vi "GEOM_CorrectAmplifiers.vi"(7 "BinCorrectionType":T1(ring), 8 "error in (no error)":errorcluster, 9 "modifiers":T6={"Binning"={"x"=1, "y"=1}, "sections"=[]} {"Binning"."y" min=1; "Binning"."x" min=1}, 10 "Amplifiers":T2[](array[typedef]) {"fliped" items=["none", "horizontal", "vertical"]; "type" items=["LL", "LR", "UL", "UR"]}) -> (0 "error out":errorcluster, 1 "NonBinnedAmplifiers":T2[](array[typedef]) {"fliped" items=["none", "horizontal", "vertical"]; "type" items=["LL", "LR", "UL", "UR"]}, 2 "BinnedAmplifiers":T2[](array[typedef]) {"fliped" items=["none", "horizontal", "vertical"]; "type" items=["LL", "LR", "UL", "UR"]})   [LabVIEW 2016]
uses:
  GEOM_AmpModifiers.ctl
  GEOM_Binning.ctl
  GEOM_Moifier.ctl
  GEOM_Amplifier.ctl
  GEOM_AmpType.ctl
  GEOM_ROI.ctl
  GEOM_Coords.ctl
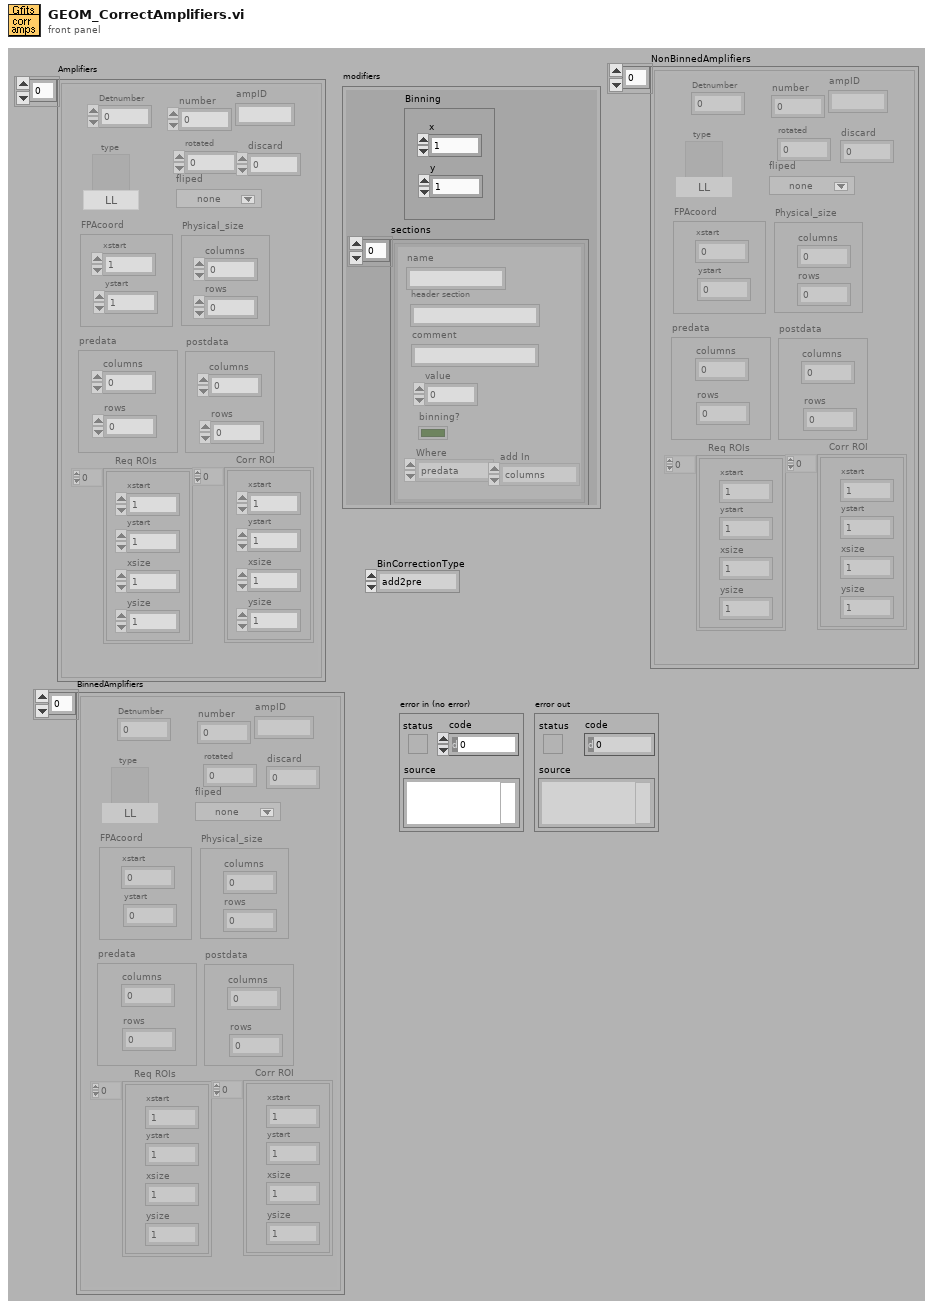
[diagram p1: front panel]
types:
  T1 = enum16{"add2pre", "add2post", "add2data", "none"}
  T2 = typedef "GEOM_Amplifier.ctl" = cluster{"number":i32, "type":T3, "rotated":i16, "fliped":u16, "FPAcoord":cluster{"xstart":i32, "ystart":i32}, "Physical_size":cluster{"columns":i32, "rows":i32}, "predata":cluster{"columns":i32, "rows":i32}, "postdata":cluster{"columns":i32, "rows":i32}, "Req ROIs":T4, "Corr ROI":T4, "Detnumber":i32, "ampID":string, "discard":i32}
  T3 = typedef "GEOM_AmpType.ctl" = u16
  T4 = typedef "GEOM_ROI.ctl" = T5[]
  T5 = typedef "GEOM_Coords.ctl" = cluster{"xstart":u32, "ystart":u32, "xsize":u32, "ysize":u32}
  T6 = typedef "GEOM_AmpModifiers.ctl" = cluster{"Binning":T7, "sections":T8[]}
  T7 = typedef "GEOM_Binning.ctl" = cluster{"x":u32, "y":u32}
  T8 = typedef "GEOM_Moifier.ctl" = cluster{"name":string, "header section":string, "comment":string, "value":i32, "binning?":bool, "Where":enum16{"predata", "postdata"}, "add In":enum16{"columns", "rows", "none"}}
  T9 = cluster{"xstart":i32, "ystart":i32, "columns":i32, "rows":i32}
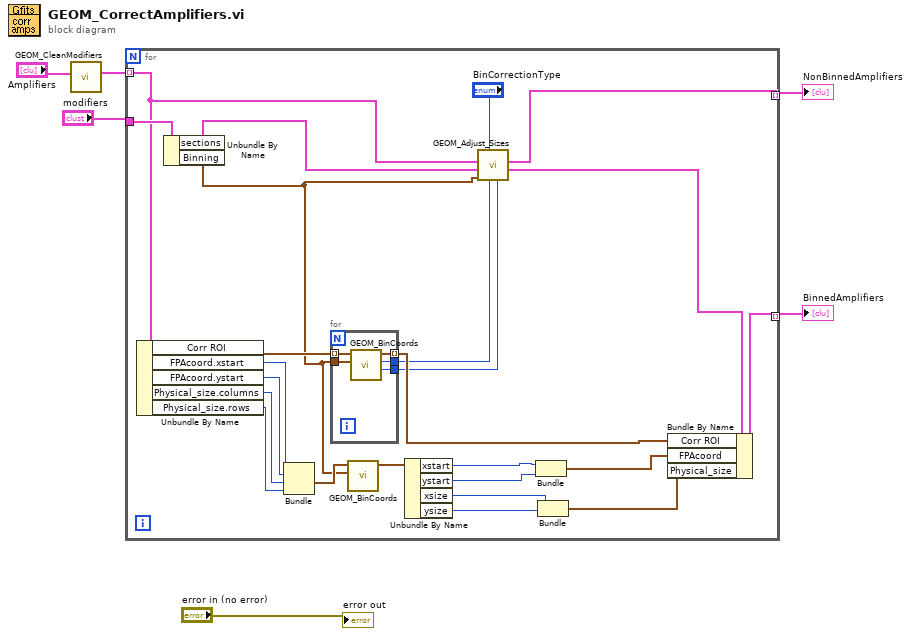
[diagram p0: block diagram]
diagram:
  n1 = call "GEOM_CleanModifiers.vi"("amplifiers in"="Amplifiers") -> ("amplifiers out"=w3:T2[])  [unwired: 10 out]
  n2 = for {
    tunnel: w3 -> [w13] mode=indexing
    tunnel: "modifiers" -> [w27]
    tunnel: [w8] -> w2 mode=indexing
    tunnel: [w28] -> w1 mode=indexing
    n3 = Unbundle By Name(w13) -> ("Corr ROI"=w30:T4, "FPAcoord.xstart"=w26:i32, "FPAcoord.ystart"=w25:i32, "Physical_size.columns"=w19:i32, "Physical_size.rows"=w18:i32)
    n4 = Unbundle By Name(w27) -> ("sections"=w12:T8[], "Binning"=w11:T7)
    n5 = Bundle("xstart"=w26, "ystart"=w25, "columns"=w19, "rows"=w18) -> (w24:T9)  [unwired: 1 out]
    n6 = for {
      tunnel: w30 -> [w35] mode=indexing
      tunnel: w11 -> [w34]
      tunnel: [w33] -> w29 mode=indexing
      tunnel: [w32] -> w10
      tunnel: [w31] -> w9
      n7 = call "GEOM_BinCoords.vi"("Binning"=w34, "coords"=w35) -> ("remaining Y"=w31:i32, "remainingX"=w32:i32, "binnedcoords"=w33:T5)  [unwired: 7 out]
    }
    n8 = call "GEOM_BinCoords.vi"("Binning"=w11, "coords"=w24) -> ("binnedcoords"=w23:T5)  [unwired: 9 out]
    n9 = Unbundle By Name(w23) -> ("xstart"=w22:u32, "ystart"=w21:u32, "xsize"=w17:u32, "ysize"=w16:u32)
    n10 = call "GEOM_Adjust_Sizes.vi"("remaining Y"=w9, "remainingX"=w10, "BinCorrectionType"="BinCorrectionType", "Binning"=w11, "sections"=w12, "Amplifier"=w13) -> ("binned amp"=w7:T2, "non-binned amp"=w8:T2)  [unwired: 4 out]
    n11 = Bundle("xstart"=w22, "ystart"=w21) -> (w15:cluster{"xstart":u32, "ystart":u32})  [unwired: 1 out]
    n12 = Bundle("xsize"=w17, "ysize"=w16) -> (w20:cluster{"xsize":u32, "ysize":u32})  [unwired: 1 out]
    n13 = Bundle By Name(cluster=w7, "Corr ROI"=w29, "FPAcoord"=w15, "Physical_size"=w20) -> (w28:T2)
  }
  "NonBinnedAmplifiers" <- w2
  "BinnedAmplifiers" <- w1
  "error out" <- "error in (no error)"
